vi "CamTestGetEvntsResponse.vi"(8 "error in (no error)":errorcluster, 10 "CameraTestingEvnt":T1, 11 "CameraTestingUI in":refnum<class "CameraTestingUI.lvclass">) -> (0 "error out":errorcluster, 3 "CameraTestingUI out":refnum<class "CameraTestingUI.lvclass">)   [LabVIEW 2020, in "CameraTestingUI.lvlib" / "CameraTestingUI.lvclass"]
uses:
  CameraTestingUI.lvclass
  ICameraTesting/ICameraTesting/TypeDef/Events.ctl
  Camera/ICamera/ICamera/TypeDef/SnapInfo.ctl
  ICameraTesting/ICameraTesting/TypeDef/FrameRateValReceived.ctl
  ICameraTesting/ICameraTesting/TypeDef/ImgTypeValReceived.ctl
  ICameraTesting/ICameraTesting/TypeDef/ResolutionValReceived.ctl
  ICameraTesting/ICameraTesting/TypeDef/VideoOptCodesUpdated.ctl
  ICameraTesting/ICameraTesting/TypeDef/VideoOptionsInfo.ctl
  ICameraTesting/ICameraTesting/TypeDef/StatusUpdated.ctl
  ICameraTesting/ICameraTesting/TypeDef/StatusRecord.ctl
  ICameraTesting/ICameraTesting/TypeDef/VideoBufferUpdate.ctl
  CameraTestingUI.lvclass/CameraTestingUI.ctl
  <vilib>/event_ctls.llb/usereventprio.ctl
  Camera/ICamera/ICamera/ICamera.lvclass
  ICameraTesting/ICameraTesting/ICameraTesting.lvclass
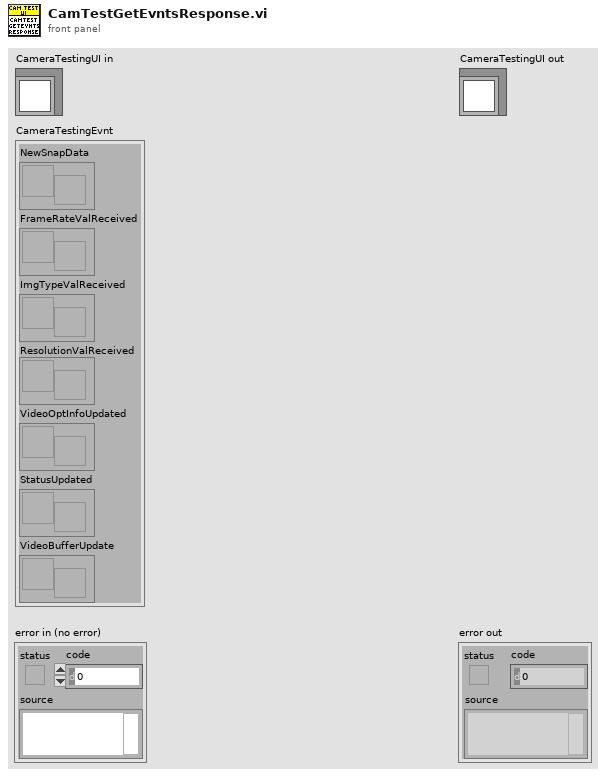
[diagram p1: front panel]
types:
  T1 = typedef "ICameraTesting.lvlib/ICameraTesting.lvclass/Events.ctl" = cluster{"NewSnapData":refnum<user-event>, "FrameRateValReceived":T2, "ImgTypeValReceived":T3, "ResolutionValReceived":T4, "VideoOptInfoUpdated":T5, "StatusUpdated":T6, "VideoBufferUpdate":T7}
  T2 = typedef "ICameraTesting.lvlib/ICameraTesting.lvclass/FrameRateValReceived.ctl" = refnum<user-event>
  T3 = typedef "ICameraTesting.lvlib/ICameraTesting.lvclass/ImgTypeValReceived.ctl" = refnum<user-event>
  T4 = typedef "ICameraTesting.lvlib/ICameraTesting.lvclass/ResolutionValReceived.ctl" = refnum<user-event>
  T5 = typedef "ICameraTesting.lvlib/ICameraTesting.lvclass/VideoOptCodesUpdated.ctl" = refnum<user-event>
  T6 = typedef "ICameraTesting.lvlib/ICameraTesting.lvclass/StatusUpdated.ctl" = refnum<user-event>
  T7 = typedef "ICameraTesting.lvlib/ICameraTesting.lvclass/VideoBufferUpdate.ctl" = refnum<user-event>
  T8 = typedef "usereventprio.ctl" = enum32{"high priority", "normal priority"}
  T9 = typedef "CameraTestingUI.lvlib/CameraTestingUI.lvclass/UpdCamTestEvntRegRef.ctl" = refnum<user-event>
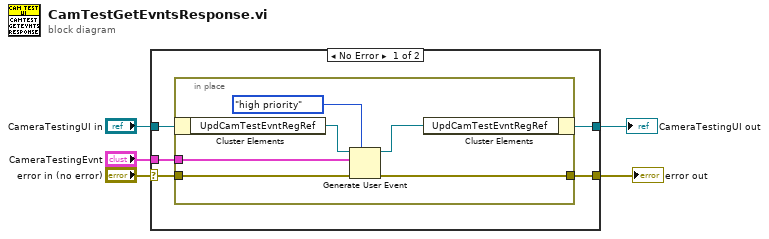
[diagram p0: block diagram]
diagram:
  n1 = case shown="No Error" "error in (no error)" {
    selector: "error in (no error)" -> [w7 w18]
    tunnel: "CameraTestingUI in" -> [w10 w17]
    tunnel: "CameraTestingEvnt" -> [w9 _]
    tunnel: [w6 w18] -> w2
    tunnel: [w8 w17] -> w1
    frame No Error {
      n2 = in-place {
        in-place-border: w9 -> [w14]
        in-place-border: w7 -> [w16]
        in-place-border: [w12] -> w6
        n3 = in-place-cluster #1(w10) -> ("UpdCamTestEvntRegRef"=w15:T9)
        n4 = Generate User Event(priority (normal)=usereventprio."high priority", user event=w15, event data cluster=w14, error in=w16) -> (user event out=w13:T9, error out=w12:errorcluster)
        n5 = in-place-cluster #1("UpdCamTestEvntRegRef"=w13) -> (w8:refnum<class "CameraTestingUI.lvclass">)
      }
    }
    frame Error {
    }
  }
  "error out" <- w2
  "CameraTestingUI out" <- w1
